vi "Apply Calibration - Slope Only.vi"(10 "slope":dbl, 11 "Waveform in":waveform(dbl)) -> (3 "Waveform out":waveform(dbl))   [LabVIEW 2020]
doc: "Use the calibration sensitivity (lbs load cell force / strain gauge volts) to scale the strain data.\n\nCalculates the mean (dc offset) of the signal and subtracts it from the strain data."
uses:
  <vilib>/measure/madcrms.llb/Basic Averaged DC-RMS for 1 Chan.vi
  <vilib>/measure/NI_MAPro.lvlib
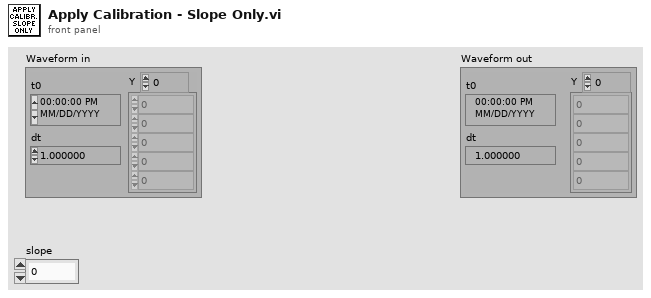
[diagram p1: front panel]
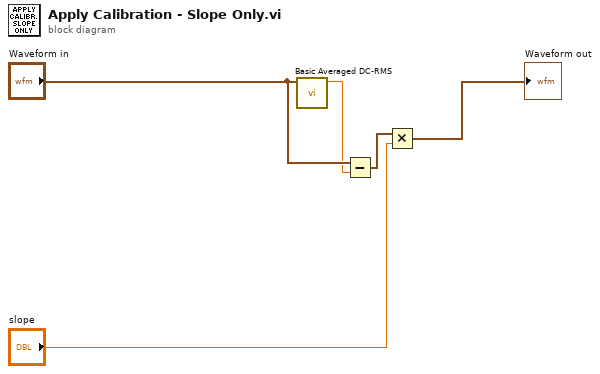
[diagram p0: block diagram]
diagram:
  n1 = call-poly <vilib>:"Basic Averaged DC-RMS.vi"("signal in"="Waveform in") -> ("DC value"=w1:dbl)  [unwired: 7 in, 3 out]
  n2 = Subtract(x="Waveform in", y=w1) -> (x-y=w3:waveform(dbl))
  n3 = Multiply(x=w3, y="slope") -> (x*y=→"Waveform out":waveform(dbl))
